vi "Escape String.vi"(10 "String":string, 11 "Serializer.PlainText in":refnum<class "Serializer.PlainText.lvclass">) -> (2 "Escaped String":string)   [LabVIEW 2013, in "OpenSerializer.lvlib" / "Serializer.PlainText.lvclass"]
uses:
  Serializer.PlainText.lvclass
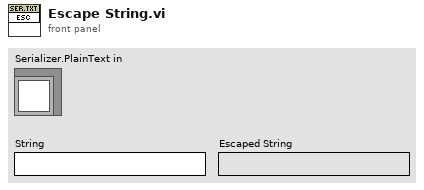
[diagram p1: front panel]
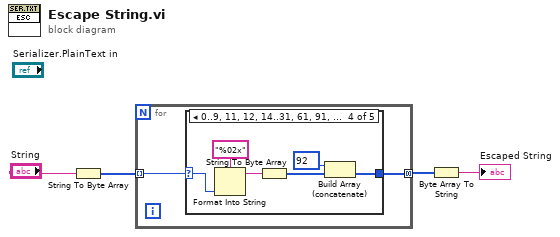
[diagram p0: block diagram]
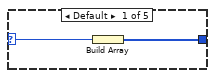
[diagram p2: hidden frame]
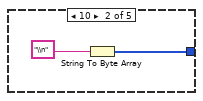
[diagram p3: hidden frame]
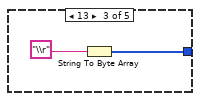
[diagram p4: hidden frame]
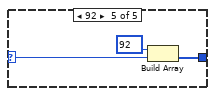
[diagram p5: hidden frame]
diagram:
  n1 = String To Byte Array(string="String") -> (unsigned byte array=w4:u8[])
  n2 = for {
    tunnel: w4 -> [w6] mode=indexing
    tunnel: [w5] -> w3 mode=concatenating
    n3 = case shown="0..9, 11, 12, 14..31, 61, 91, 93, 254, 255" w6 {
      selector: w6 -> [w8 _ _ w17 w19]
      tunnel: [w7 w9 w11 w13 w20] -> w5
      frame Default {
        n4 = Build Array(w8) -> (w7:u8[])
      }
      frame 10 {
        n5 = String To Byte Array(string="\\n" ("replace string (\"\")")) -> (unsigned byte array=w9:u8[])
      }
      frame 13 {
        n6 = String To Byte Array(string="\\r" ("replace string (\"\")")) -> (unsigned byte array=w11:u8[])
      }
      frame 0..9, 11, 12, 14..31, 61, 91, 93, 254, 255 {
        n7 = Format Into String(format string="%02x", w17) -> (resulting string=w16:string)  [unwired: 2 in, 1 out]
        n8 = String To Byte Array(string=w16) -> (unsigned byte array=w14:u8[])
        n9 = Build Array (concatenate)(u8 92, w14) -> (w13:u8[])
      }
      frame 92 {
        n10 = Build Array(u8 92, w19) -> (w20:u8[])
      }
    }
  }
  n11 = Byte Array To String(unsigned byte array=w3) -> (string=→"Escaped String":string)
